vi "Extract Boolean Array.vi"() -> ()   [LabVIEW 2017]
panel:
  in  "Random String":string="RLR"
  out "Platform Sides":bool[](array[boolean])
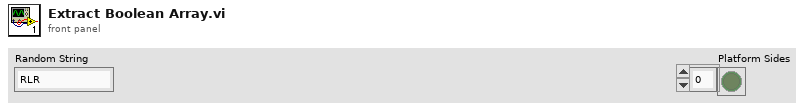
[diagram p1: front panel]
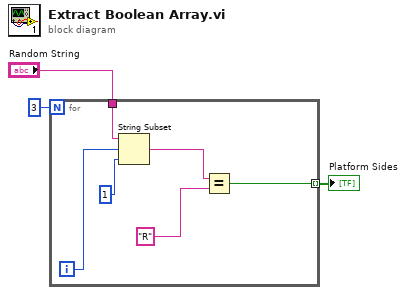
[diagram p0: block diagram]
diagram:
  n1 = for {
    N: 3 -> [_]
    tunnel: "Random String" -> [w8]
    tunnel: [w4] -> w1 mode=indexing
    i -> [w5]
    n2 = String Subset(string=w8, offset (0)=w5, length (rest)=1 ("length (rest)")) -> (substring=w6:string)
    n3 = Equal?(x=w6, y="R") -> (x = y?=w4:bool)
  }
  "Platform Sides" <- w1
